vi "MicroscopeControl.vi"(0 "Microscope in":refnum<class "Microscope.lvclass">) -> (4 "Microscope Out":refnum<class "Microscope.lvclass">)   [LabVIEW 2012]
uses:
  classes/Microscope.lvclass
  typedefs/ImageEvent.ctl
  typedefs/MicroscopeEvent.ctl
  variables/GlobalUI.vi
  classes/MCCPMT.lvclass
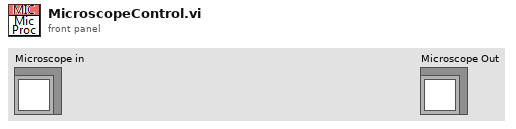
[diagram p1: front panel]
types:
  T1 = typedef "ImageEvent.ctl" = enum16{"i.Wait", "i.Acquire", "i.InitImageData", "i.ReinitImageData", "i.ReinitImageParams", "i.PreAcquire", "i.PostAcquire", "i.ClearData"}
  T2 = typedef "MicroscopeEvent.ctl" = enum16{"M.Wait", "M.RunRotation", "M.Flush", "M.Init", "M.InitStage", "M.InitImageData", "M.ReinitImageData", "M.ReinitImageParams", "M.GetSetParams", "M.InitFastHardware", "M.Pre-Acquire", "M.Acquire", "M.PostAcquire", "M.StopAcquire", "M.SetAcqStatusTrue", "M.SetAcqStatusFalse", "M.ClearImageData", "M.MoveStageDiscrete", "M.MoveStageToTarget1", "M.MoveStageToTarget2", "M.MoveStageToTarget3", "M.OpenShutters", "M.CloseShutters", "M.StartAcquireSequence", "M.ChangeParameters", "M.OpenStokes", "M.OpenPump", "M.RunSW"}
  T3 = typedef "HWsettings.ctl" = cluster{"Galvo Channels":tag, "Detector Channels":tag, "Galvo Trigger":tag, "Shutter Lines":tag[], "Max Acquisition Rate":dbl, "Recommended Acquisition Rate":dbl, "Galvo Write Rate":dbl, "Max Timebase Frequency (Hz)":dbl, "MCC Shutter Lines":refnum<k21>[], "Detector Task":refnum<k21>, "Shutter Tasks":refnum<k21>[], "Galvo Task":refnum<k21>, "Digital Image Multiplier":dbl[]}
  T4 = typedef "Scan Parameters.ctl" = cluster{"x pixels":i32, "x voltage min":dbl, "x voltage max":dbl, "y voltage min":dbl, "y voltage max":dbl, "fill frac":dbl, "Zoom":dbl, "BiDi":bool, "scan rate (ms/line)":dbl}
  T5 = typedef "Stage Parameters.ctl" = cluster{"Scan Mode":T6, "Start position mm":dbl, "End position mm":dbl, "Velocity um/sec (continuous)":dbl, "Step size microns (discrete)":dbl, "Frames to grab (grab)":i32}
  T6 = typedef "ScanMode.ctl" = enum16{"None", "Continuous", "Point Scan (CH3 cursor)", "Point Scan Move (CH3 cursor)", "Grab", "Grab Move Stage", "Grab Move Z-stage", "Cont. Move Z-stage", "Spec Move Stage", "Spec Move Cont", "Surf Calib"}
  T7 = typedef "SyncAlgo.ctl" = cluster{"Pixels/sec":dbl, "Pixel Dwell Time (us)":dbl, "Fill Factor":dbl, "Flyback Pixels":dbl, "Lines/sec":dbl, "Galvo Write rate":dbl, "Galvo Timebase divisor":i32, "total pixels per line":dbl, "Samples to Average":dbl, "Trash Samples":dbl, "Actual samples to Read per Line":dbl, "Detector Read rate":dbl, "Detector Timebase divisor":i32}
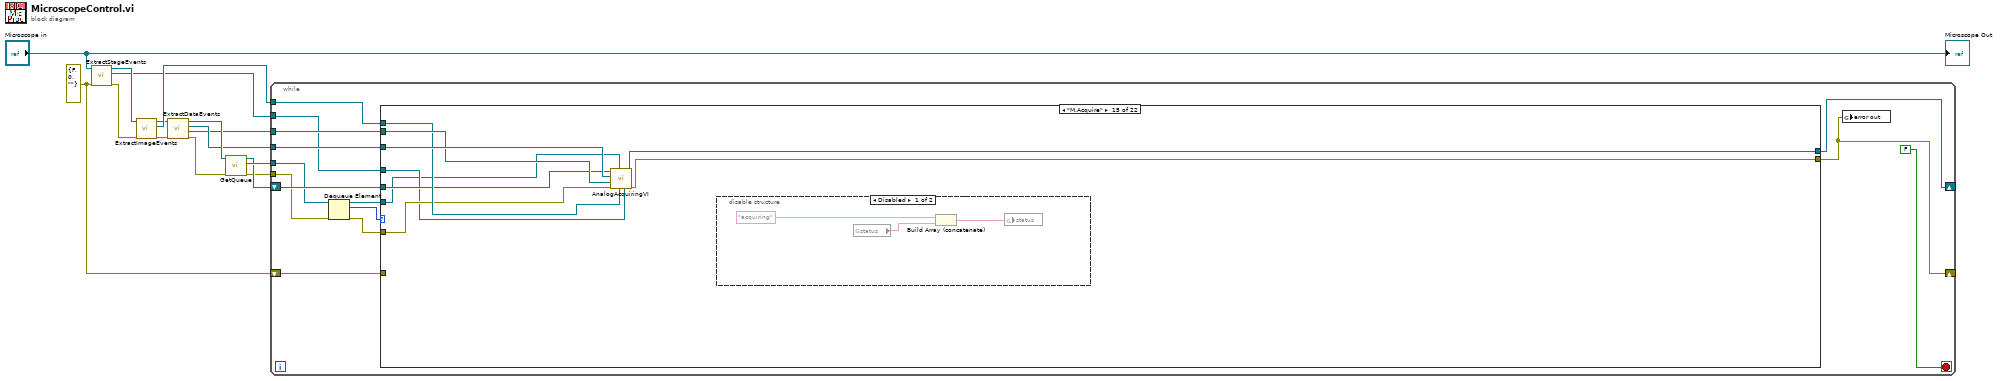
[diagram p0: block diagram]
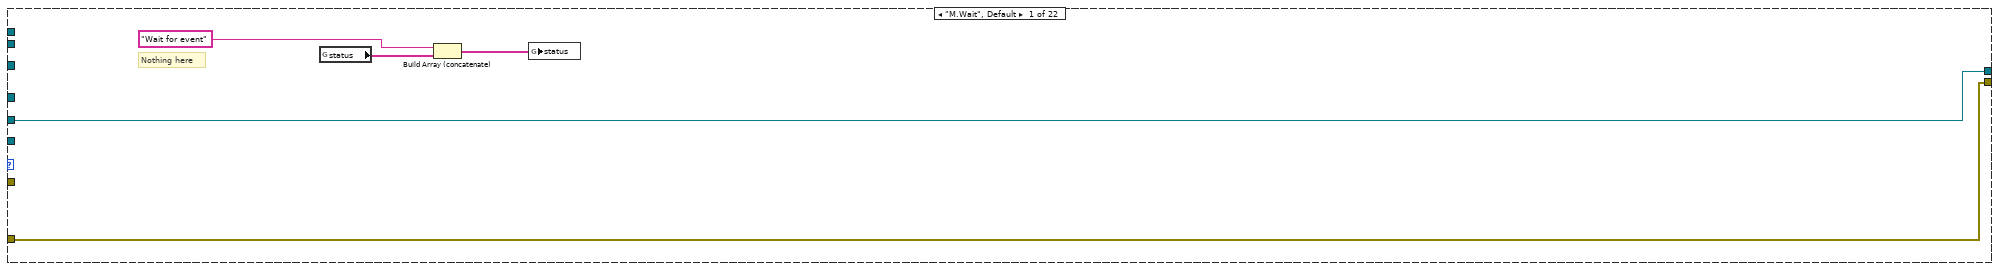
[diagram p2: hidden frame]
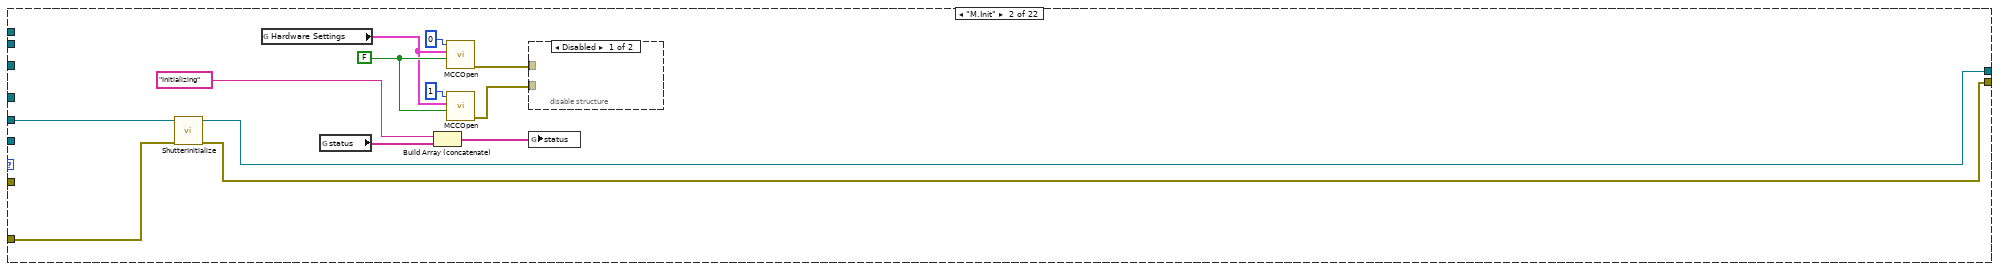
[diagram p3: hidden frame]
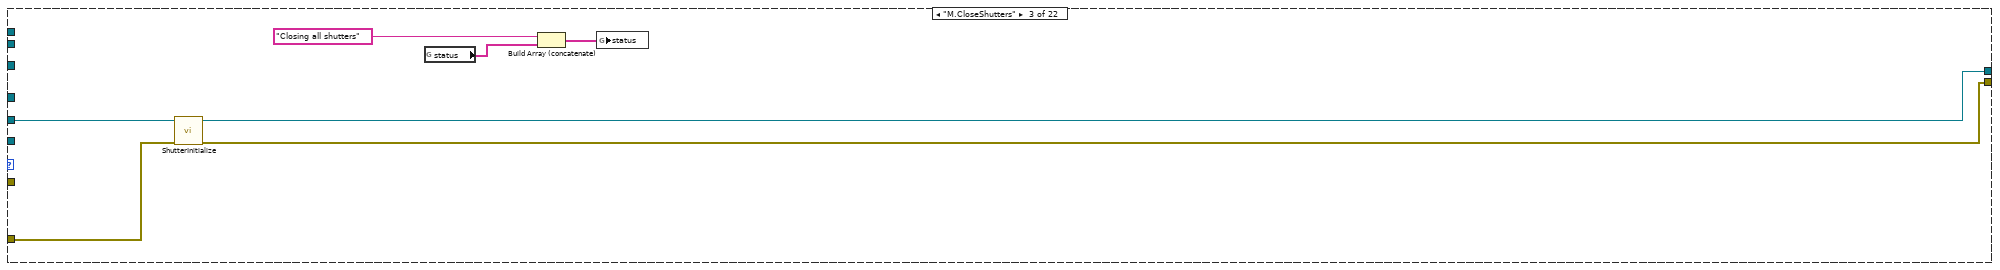
[diagram p5: hidden frame]
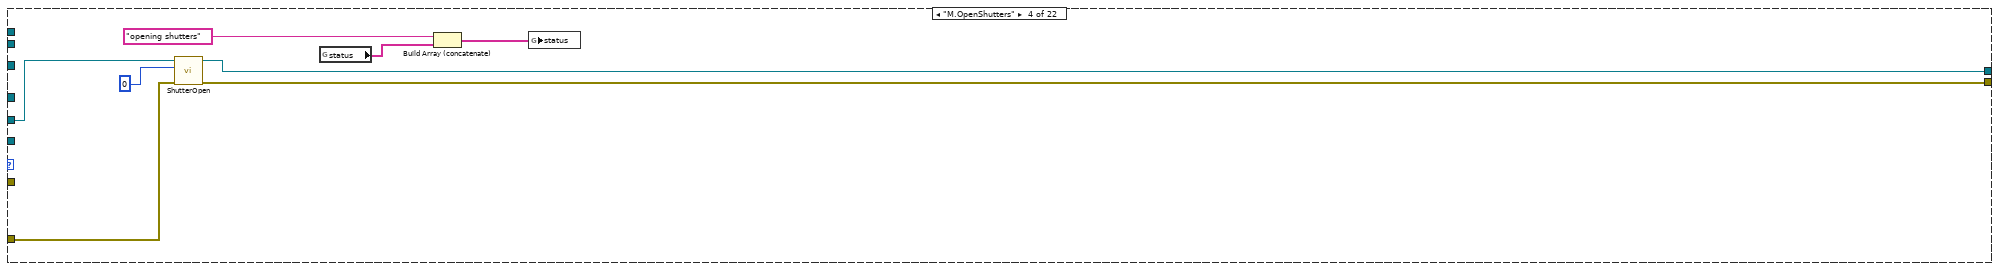
[diagram p6: hidden frame]
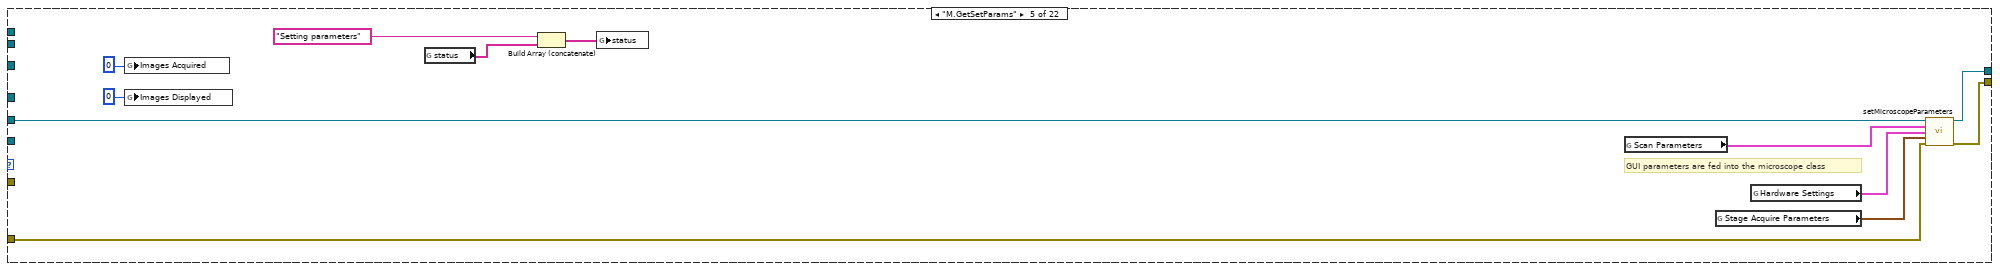
[diagram p7: hidden frame]
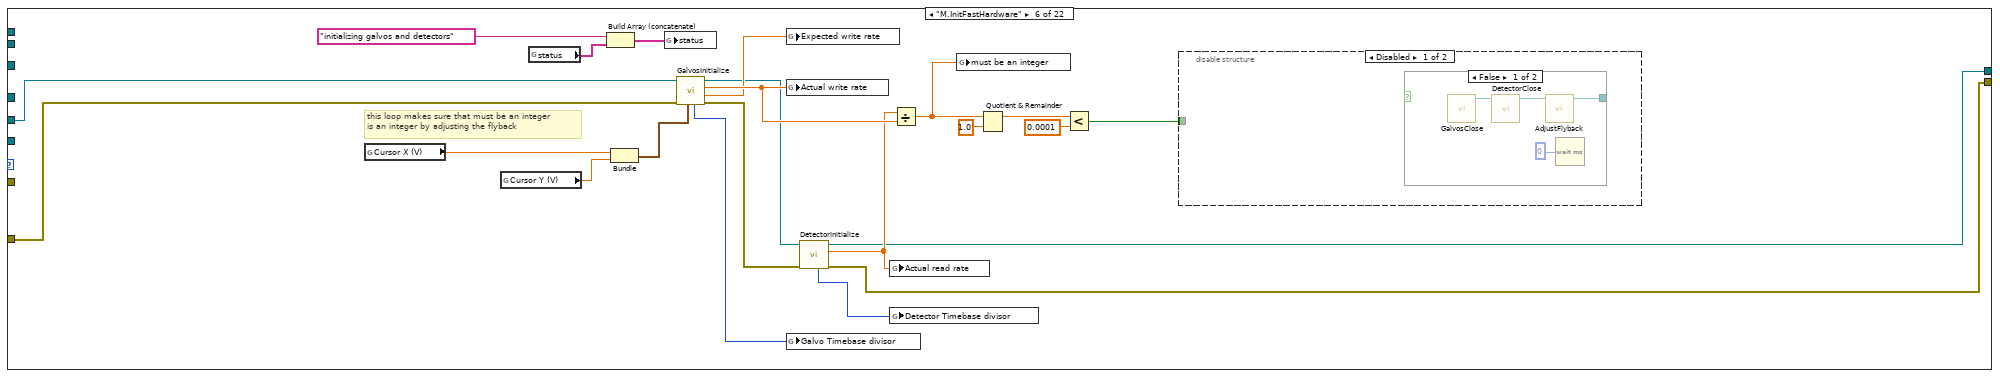
[diagram p8: hidden frame]
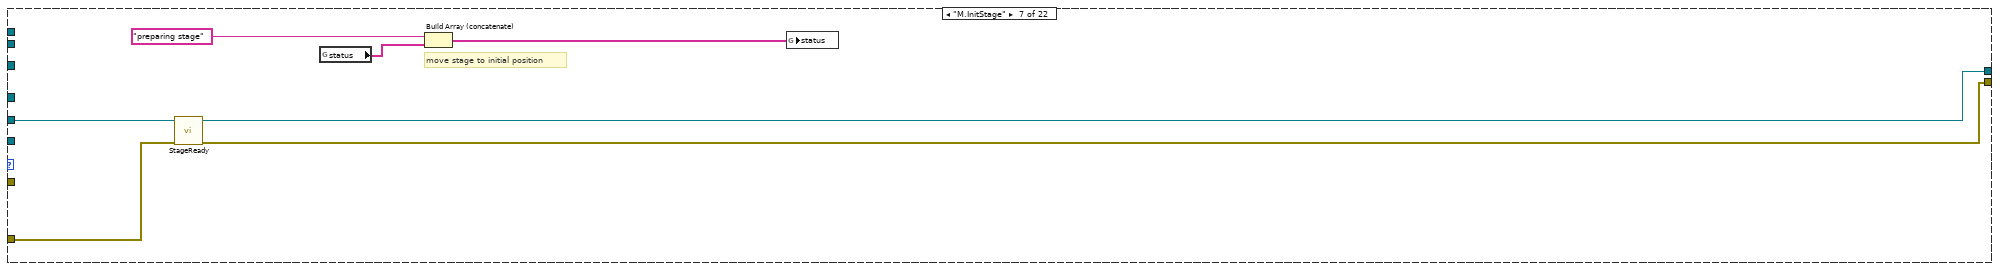
[diagram p11: hidden frame]
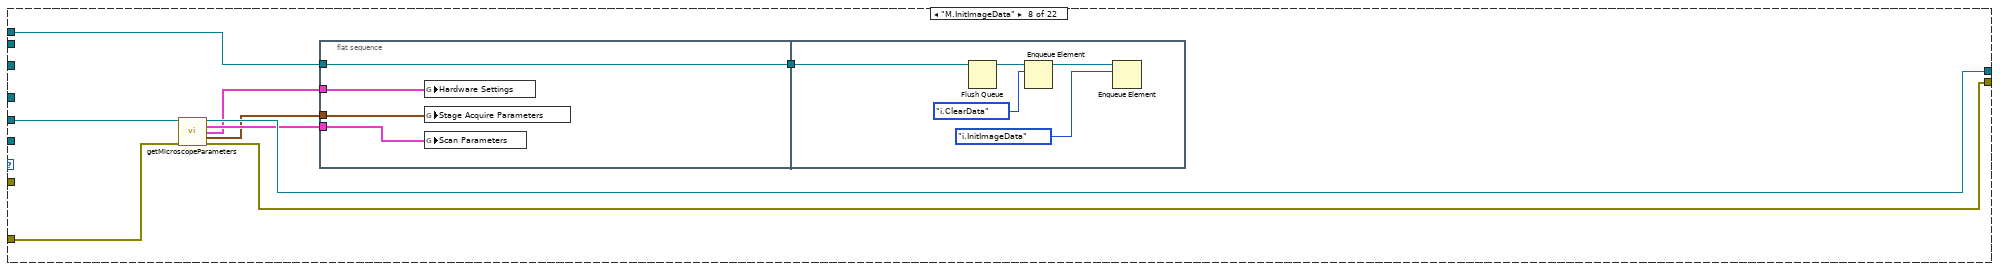
[diagram p12: hidden frame]
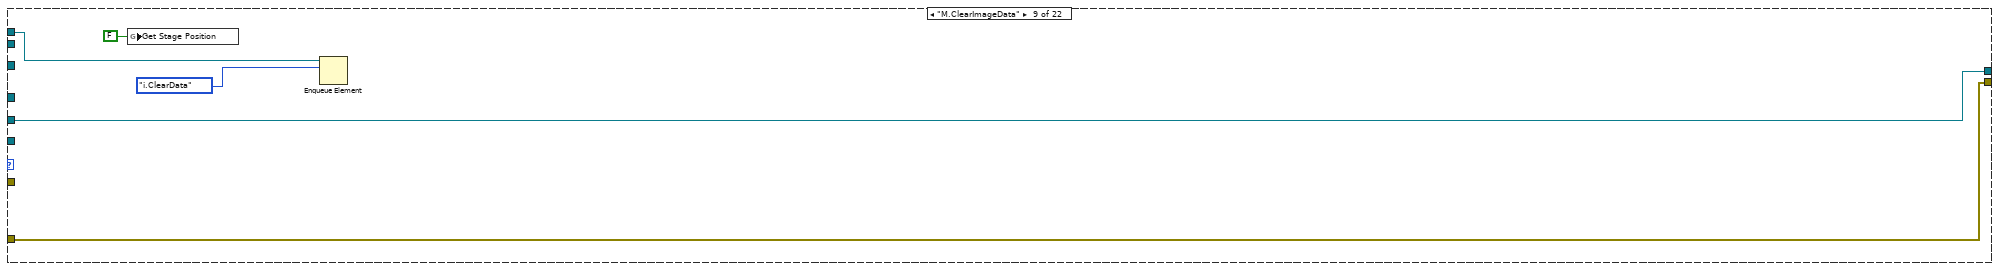
[diagram p13: hidden frame]
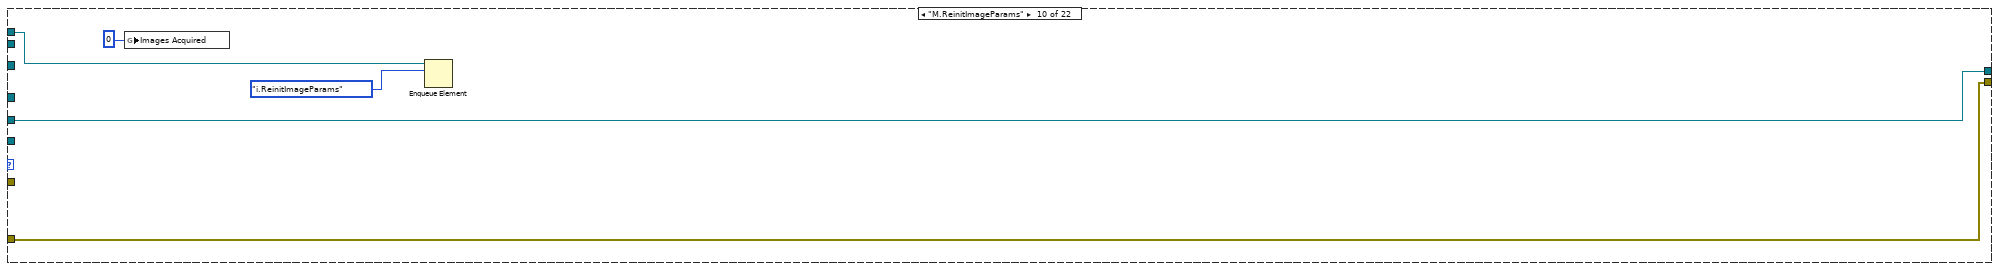
[diagram p14: hidden frame]
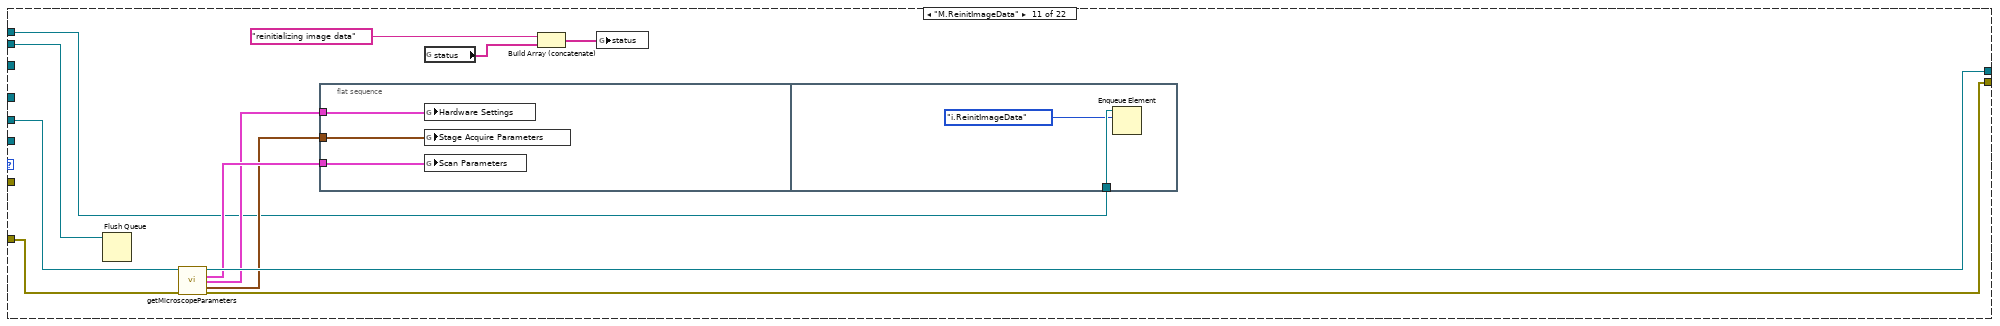
[diagram p15: hidden frame]
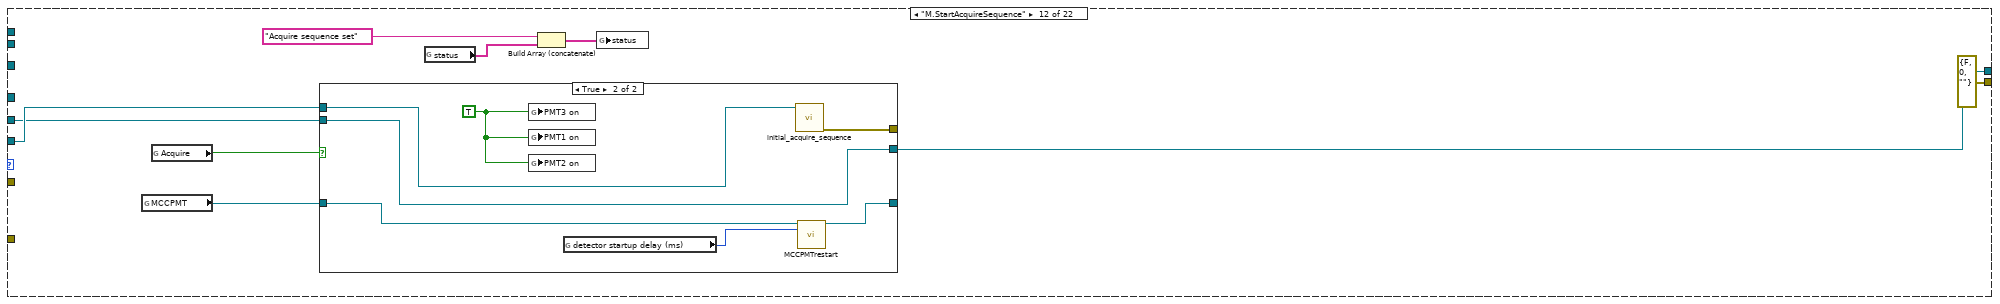
[diagram p16: hidden frame]
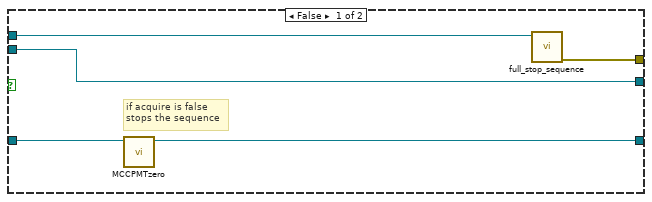
[diagram p17: hidden frame]
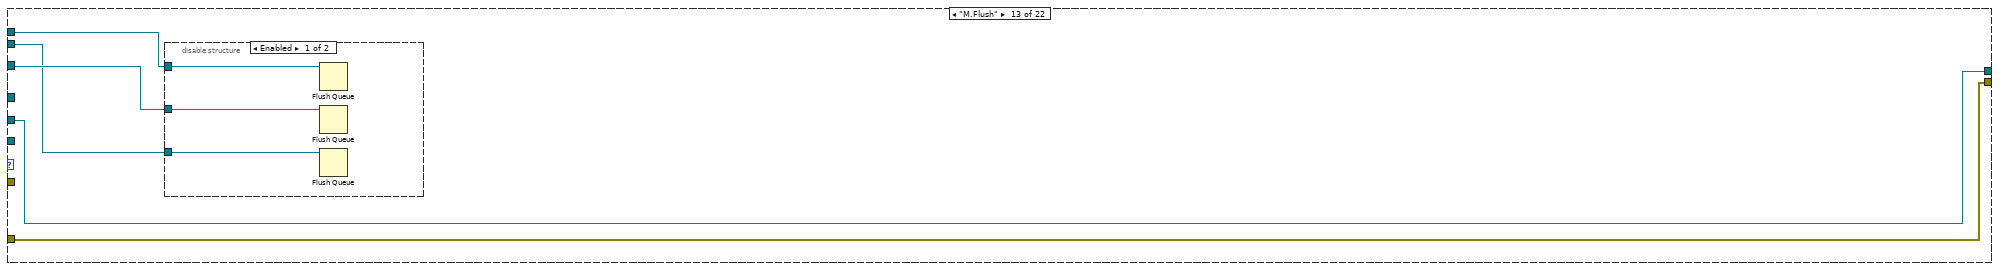
[diagram p18: hidden frame]
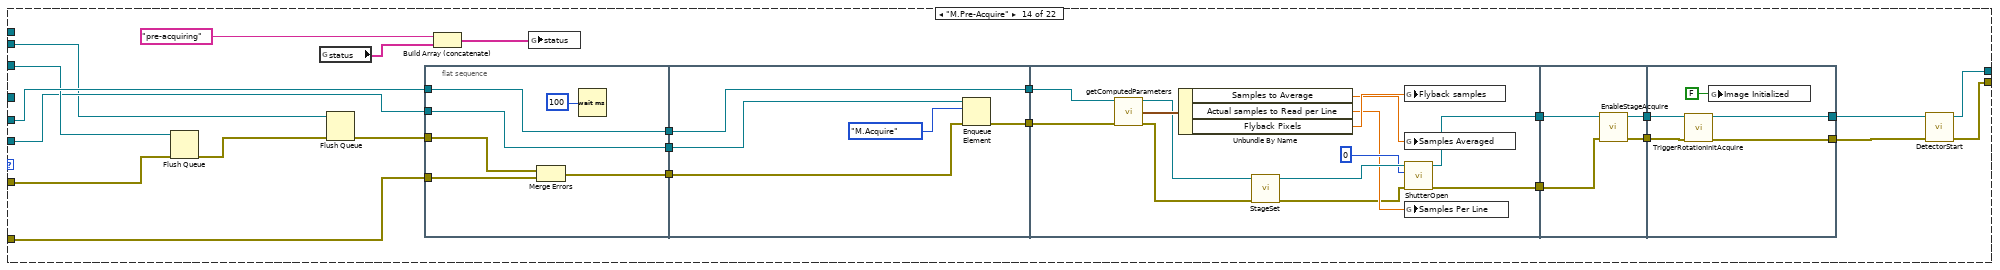
[diagram p20: hidden frame]
diagram:
  w2 = errorcluster {"status"=FALSE, "code"=0, "source"=""} ("error out")
  n1 = call "ExtractStageEvents.vi"("error in (no error)"=w2, "Microscope in"="Microscope in") -> ("error out"=w4:errorcluster, "Stage events"=w1:refnum<queue>, "Microscope out"=w5:refnum<class "Microscope.lvclass">)  [unwired: 6 in, 1 out]
  n2 = call "ExtractImageEvents.vi"("error in (no error)"=w4, "Microscope in"=w5) -> ("error out"=w6:errorcluster, "Image events"=w13:refnum<queue>, "Microscope out"=w12:refnum<class "Microscope.lvclass">)  [unwired: 7 in]
  n3 = call "ExtractDataEvents.vi"("error in (no error)"=w6, "Microscope in"=w12) -> ("error out"=w7:errorcluster, "Raw Data"=w9:refnum<queue>, "X Data"=w10:refnum<queue>, "Microscope out"=w11:refnum<class "Microscope.lvclass">)  [unwired: 6 in]
  n4 = call "GetQueue.vi"("error in (no error)"=w7, "Microscope in"=w11) -> ("error out"=w8:errorcluster, "Microscope events"=w15:refnum<queue>, "Microscope out"=w14:refnum<class "Microscope.lvclass">)  [unwired: 7 in]
  n5 = while {
    shift-right: [w28] -> _
    shift-left: w14 -> [w29]
    shift-right: [w19] -> _
    shift-left: w2 -> [w21]
    tunnel: w15 -> [w20]
    tunnel: w9 -> [w24]
    tunnel: w13 -> [w23]
    tunnel: w10 -> [w22]
    tunnel: w8 -> [w17]
    tunnel: w1 -> [w16]
    stop <- FALSE stop-if-true
    n6 = Dequeue Element(queue=w20, error in (no error)=w17) -> (queue out=w27:refnum<queue>, element=w26:T2, error out=w18:errorcluster)  [unwired: 1 in, 1 out]
    n7 = case shown="\"M.Acquire\"" w26 {
      tunnel: w29 -> [w34 w45 w52 w61 w74 w88 w103 w117 w130 w136 w148 w156 w179 w206 w245 w267 w282 w291 w299 w306 w313 w321]
      tunnel: [w34 w47 w54 w60 w64 w75 w105 w116 w130 w136 w147 w155 w179 w204 w240 w258 w269 w290 w299 w306 w309 w314] -> w28
      tunnel: [w33 w46 w53 w59 w63 w95 w104 w115 w129 w135 w145 errorcluster {"status"=FALSE, "code"=0, "source"=""} ("error out") w178 w205 w241 w257 w271 w288 w300 w307 w308 w315] -> w19
      tunnel: w21 -> [w33 w44 w51 w58 w65 w96 w102 w114 w129 w135 w146 _ w178 w203 _ w268 w280 w289 w300 w307 w312 w320]
      tunnel: w27 -> [_ _ _ _ _ _ _ _ _ _ _ w162 _ w201 w242 w264 _ _ _ _ _ _]
      tunnel: w24 -> [_ _ _ _ _ _ _ _ _ _ w140 _ w176 w200 w247 _ _ _ _ _ _ _]
      tunnel: w23 -> [_ _ _ _ _ _ _ w110 w131 w134 w141 _ w175 _ w246 w263 _ _ _ _ _ _]
      tunnel: w22 -> [_ _ _ _ _ _ _ _ _ _ _ _ w177 w202 w248 _ _ _ _ _ _ _]
      tunnel: w18 -> [_ _ _ _ _ _ _ _ _ _ _ _ _ w192 w244 _ _ _ _ _ _ _]
      tunnel: w16 -> [_ _ _ _ _ _ _ _ _ _ _ _ _ _ w243 _ w270 _ _ _ _ _]
      frame "M.Wait", Default {
        # "Nothing here"
        n8 = global read "GlobalUI.vi" "status"() -> (w32:string[])
        n9 = Build Array (concatenate)("Wait for event" ("status"), w32) -> (w31:string[])
        n10 = global write "GlobalUI.vi" "status"(w31) -> ()
      }
      frame "M.Init" {
        w41 = FALSE ("Open")
        n11 = call "ShutterInitialize.vi"("error in (no error)"=w44, "Microscope in"=w45) -> ("error out"=w46:errorcluster, "Microscope out"=w47:refnum<class "Microscope.lvclass">)  [unwired: 8 in]
        n12 = global read "GlobalUI.vi" "Hardware Settings"() -> (w37:T3)
        n13 = global read "GlobalUI.vi" "status"() -> (w40:string[])
        n14 = Build Array (concatenate)("Initializing" ("status"), w40) -> (w39:string[])
        n15 = call "MCCOpen.vi"("Open"=w41, "Hardware Settings"=w37, "index"=0) -> ("error out"=w36:errorcluster)  [unwired: 8 in]
        n16 = call "MCCOpen.vi"("Open"=w41, "Hardware Settings"=w37, "index"=1) -> ("error out"=w35:errorcluster)  [unwired: 8 in]
        n17 = disable-structure shown="Disabled" {
          disable-tunnel: w36 -> [_ _]
          disable-tunnel: w35 -> [_ _]
          frame Disabled {
          }
          frame Enabled {
          }
        }
        n18 = global write "GlobalUI.vi" "status"(w39) -> ()
      }
      frame "M.CloseShutters" {
        n19 = call "ShutterInitialize.vi"("error in (no error)"=w51, "Microscope in"=w52) -> ("error out"=w53:errorcluster, "Microscope out"=w54:refnum<class "Microscope.lvclass">)  [unwired: 8 in]
        n20 = global read "GlobalUI.vi" "status"() -> (w50:string[])
        n21 = Build Array (concatenate)("Closing all shutters" ("status"), w50) -> (w48:string[])
        n22 = global write "GlobalUI.vi" "status"(w48) -> ()
      }
      frame "M.OpenShutters" {
        n23 = call "ShutterOpen.vi"("error in (no error)"=w58, "Shutter number"=0, "Microscope in"=w61) -> ("error out"=w59:errorcluster, "Microscope out"=w60:refnum<class "Microscope.lvclass">)  [unwired: 7 in]
        n24 = global read "GlobalUI.vi" "status"() -> (w57:string[])
        n25 = Build Array (concatenate)("opening shutters" ("status"), w57) -> (w56:string[])
        n26 = global write "GlobalUI.vi" "status"(w56) -> ()
      }
      frame "M.GetSetParams" {
        # "GUI parameters are fed into the microscope class"
        n27 = global write "GlobalUI.vi" "Images Acquired"(0 ("images grabbed")) -> ()
        n28 = global write "GlobalUI.vi" "Images Displayed"(0 ("Frames grabbed")) -> ()
        n29 = global read "GlobalUI.vi" "status"() -> (w69:string[])
        n30 = Build Array (concatenate)("Setting parameters" ("status"), w69) -> (w68:string[])
        n31 = global write "GlobalUI.vi" "status"(w68) -> ()
        n32 = global read "GlobalUI.vi" "Scan Parameters"() -> (w67:T4)
        n33 = global read "GlobalUI.vi" "Stage Acquire Parameters"() -> (w70:T5)
        n34 = global read "GlobalUI.vi" "Hardware Settings"() -> (w66:T3)
        n35 = call "setMicroscopeParameters.vi"("Microscope in"=w74, "Scan Parameters"=w67, "Hardware Settings"=w66, "Stage Acquire Parameters"=w70, "error in (no error)"=w65) -> ("Microscope out"=w64:refnum<class "Microscope.lvclass">, "error out"=w63:errorcluster)  [unwired: 9 in]
      }
      frame "M.InitFastHardware" {
        # "this loop makes sure that must be an integer\nis an integer by adjusting the flyback"
        n36 = global read "GlobalUI.vi" "Cursor X (V)"() -> (w91:dbl)
        n37 = global read "GlobalUI.vi" "Cursor Y (V)"() -> (w90:dbl)
        n38 = global read "GlobalUI.vi" "status"() -> (w94:string[])
        n39 = Build Array (concatenate)("initializing galvos and detectors" ("status"), w94) -> (w93:string[])
        n40 = Bundle("Cursor X (V)"=w91, "Cursor Y (V)"=w90) -> (w89:cluster{"Cursor X (V)":dbl, "Cursor Y (V)":dbl})  [unwired: 1 in]
        n41 = global write "GlobalUI.vi" "status"(w93) -> ()
        n42 = call "GalvosInitialize.vi"("Cursor Position (V)"=w89, "error in (no error)"=w96, "Microscope in"=w88) -> ("error out"=w87:errorcluster, "Galvo Write Rate"=w85:dbl, "actual write rate"=w86:dbl, "Microscope out"=w83:refnum<class "Microscope.lvclass">, "Galvo Timebase divisor"=w84:i32)  [unwired: 4 in]
        n43 = global write "GlobalUI.vi" "Expected write rate"(w85) -> ()
        n44 = global write "GlobalUI.vi" "Actual write rate"(w86) -> ()
        n45 = global write "GlobalUI.vi" "Galvo Timebase divisor"(w84) -> ()
        n46 = call "DetectorInitialize.vi"("error in (no error)"=w87, "Microscope in"=w83) -> ("error out"=w95:errorcluster, "Actual read rate"=w82:dbl, "Microscope out"=w75:refnum<class "Microscope.lvclass">, "Detector Timebase divisor"=w81:i32)  [unwired: 6 in]
        n47 = global write "GlobalUI.vi" "Actual read rate"(w82) -> ()
        n48 = global write "GlobalUI.vi" "Detector Timebase divisor"(w81) -> ()
        n49 = Divide(x=w82, y=w86) -> (x/y=w80:dbl)
        n50 = global write "GlobalUI.vi" "must be an integer"(w80) -> ()
        n51 = Quotient & Remainder(x=w80, y=1.0) -> (x-y*floor(x/y)=w77:dbl)  [unwired: 1 out]
        n52 = Less?(x=w77, y=0.0001) -> (x < y?=w76:bool)
        n53 = disable-structure shown="Disabled" {
          disable-tunnel: w76 -> [w97 _]
          frame Disabled {
            n54 = case shown="False" {
              selector: _ -> [_ _]
              tunnel: [w98 _] -> _
              frame False {
                n55 = call "GalvosClose.vi"() -> ("Microscope out"=w99:refnum<class "Microscope.lvclass">)  [unwired: 10 in, 1 out]
                n56 = call "DetectorClose.vi"("Microscope in"=w99) -> ("Microscope out"=w101:refnum<class "Microscope.lvclass">)  [unwired: 9 in, 1 out]
                n57 = call "AdjustFlyback.vi"("Microscope in"=w101) -> ("Microscope out"=w98:refnum<class "Microscope.lvclass">)  [unwired: 9 in, 1 out]
                n58 = Wait (ms)(milliseconds to wait=u32 0) -> ()  [unwired: 1 out]
              }
              frame True {
              }
            }
          }
          frame Enabled {
          }
        }
      }
      frame "M.InitStage" {
        # "move stage to initial position"
        n59 = call "StageReady.vi"("error in (no error)"=w102, "Microscope in"=w103) -> ("error out"=w104:errorcluster, "Microscope out"=w105:refnum<class "Microscope.lvclass">)  [unwired: 8 in]
        n60 = global read "GlobalUI.vi" "status"() -> (w107:string[])
        n61 = Build Array (concatenate)("preparing stage" ("status"), w107) -> (w108:string[])
        n62 = global write "GlobalUI.vi" "status"(w108) -> ()
      }
      frame "M.InitImageData" {
        n63 = call "getMicroscopeParameters.vi"("Microscope in"=w117, "error in (no error)"=w114) -> ("Microscope out"=w116:refnum<class "Microscope.lvclass">, "Scan Parameters"=w113:T4, "Hardware Settings"=w112:T3, "Stage Acquire Parameters"=w111:T5, "error out"=w115:errorcluster)  [unwired: 9 in]
        n64 = flat-sequence {
          tunnel: w113 -> [w119]
          tunnel: w112 -> [w120]
          tunnel: w111 -> [w118]
          tunnel: w110 -> [w121]
          tunnel: [w121] -> w109
          tunnel: w109 -> [w125]
          frame #0 {
            n65 = global write "GlobalUI.vi" "Hardware Settings"(w120) -> ()
            n66 = global write "GlobalUI.vi" "Stage Acquire Parameters"(w118) -> ()
            n67 = global write "GlobalUI.vi" "Scan Parameters"(w119) -> ()
          }
          frame #1 {
            n68 = Flush Queue(queue=w125) -> (queue out=w124:refnum<queue>)  [unwired: 1 in, 2 out]
            n69 = Enqueue Element(queue=w124, element=ImageEvent."i.ClearData") -> (queue out=w123:refnum<queue>)  [unwired: 2 in, 2 out]
            n70 = Enqueue Element(queue=w123, element=ImageEvent."i.InitImageData") -> ()  [unwired: 2 in, 3 out]
          }
        }
      }
      frame "M.ClearImageData" {
        n71 = global write "GlobalUI.vi" "Get Stage Position"(FALSE ("Get Stage Position")) -> ()
        n72 = Enqueue Element(queue=w131, element=ImageEvent."i.ClearData") -> ()  [unwired: 2 in, 3 out]
      }
      frame "M.ReinitImageParams" {
        n73 = global write "GlobalUI.vi" "Images Acquired"(0 ("Dgrabbed")) -> ()
        n74 = Enqueue Element(queue=w134, element=ImageEvent."i.ReinitImageParams") -> ()  [unwired: 2 in, 3 out]
      }
      frame "M.ReinitImageData" {
        n75 = Flush Queue(queue=w140) -> ()  [unwired: 1 in, 3 out]
        n76 = call "getMicroscopeParameters.vi"("Microscope in"=w148, "error in (no error)"=w146) -> ("Microscope out"=w147:refnum<class "Microscope.lvclass">, "Scan Parameters"=w144:T4, "Hardware Settings"=w143:T3, "Stage Acquire Parameters"=w142:T5, "error out"=w145:errorcluster)  [unwired: 9 in]
        n77 = flat-sequence {
          tunnel: w144 -> [w150]
          tunnel: w143 -> [w151]
          tunnel: w142 -> [w149]
          tunnel: w141 -> [w153]
          frame #0 {
            n78 = global write "GlobalUI.vi" "Hardware Settings"(w151) -> ()
            n79 = global write "GlobalUI.vi" "Stage Acquire Parameters"(w149) -> ()
            n80 = global write "GlobalUI.vi" "Scan Parameters"(w150) -> ()
          }
          frame #1 {
            n81 = Enqueue Element(queue=w153, element=ImageEvent."i.ReinitImageData") -> ()  [unwired: 2 in, 3 out]
          }
        }
        n82 = global read "GlobalUI.vi" "status"() -> (w139:string[])
        n83 = Build Array (concatenate)("reinitializing image data" ("status"), w139) -> (w138:string[])
        n84 = global write "GlobalUI.vi" "status"(w138) -> ()
      }
      frame "M.StartAcquireSequence" {
        n85 = global read "GlobalUI.vi" "MCCPMT"() -> (w157:refnum<class "MCCPMT.lvclass">)
        n86 = global read "GlobalUI.vi" "Acquire"() -> (w158:bool)
        n87 = case shown="True" w158 {
          tunnel: [w167 w174] -> _
          tunnel: [w166 w173] -> _
          tunnel: w157 -> [w165 w172]
          tunnel: w162 -> [w164 w168]
          tunnel: w156 -> [w163 w169]
          tunnel: [w163 w169] -> w155
          frame False {
            # "if acquire is false\nstops the sequence"
            n88 = call "MCCPMTzero.vi"("MCCPMT in"=w165) -> ("MCCPMT out"=w166:refnum<class "MCCPMT.lvclass">)  [unwired: 9 in, 1 out]
            n89 = call "full_stop_sequence.vi"("Queue in"=w164) -> ("error out"=w167:errorcluster)  [unwired: 9 in, 1 out]
          }
          frame True {
            w171 = TRUE ("PMT2 on")
            n90 = global write "GlobalUI.vi" "PMT3 on"(w171) -> ()
            n91 = global write "GlobalUI.vi" "PMT1 on"(w171) -> ()
            n92 = global write "GlobalUI.vi" "PMT2 on"(w171) -> ()
            n93 = global read "GlobalUI.vi" "detector startup delay (ms)"() -> (w170:u32)
            n94 = call "initial_acquire_sequence.vi"("Queue in"=w168) -> ("error out"=w174:errorcluster)  [unwired: 9 in, 1 out]
            n95 = call "MCCPMTrestart.vi"("MCCPMT in"=w172, "milliseconds to wait"=w170) -> ("MCCPMT out"=w173:refnum<class "MCCPMT.lvclass">)  [unwired: 9 in, 4 out]
          }
        }
        n96 = global read "GlobalUI.vi" "status"() -> (w161:string[])
        n97 = Build Array (concatenate)("Acquire sequence set" ("status"), w161) -> (w159:string[])
        n98 = global write "GlobalUI.vi" "status"(w159) -> ()
      }
      frame "M.Flush" {
        n99 = disable-structure shown="Enabled" {
          disable-tunnel: w177 -> [w182 _]
          disable-tunnel: w176 -> [w181 _]
          disable-tunnel: w175 -> [w180 _]
          frame Enabled {
            n100 = Flush Queue(queue=w180) -> ()  [unwired: 1 in, 3 out]
            n101 = Flush Queue(queue=w182) -> ()  [unwired: 1 in, 3 out]
            n102 = Flush Queue(queue=w181) -> ()  [unwired: 1 in, 3 out]
          }
          frame Disabled {
          }
        }
      }
      frame "M.Pre-Acquire" {
        n103 = Flush Queue(queue=w202, error in (no error)=w192) -> (error out=w193:errorcluster)  [unwired: 2 out]
        n104 = global read "GlobalUI.vi" "status"() -> (w199:string[])
        n105 = Flush Queue(queue=w200, error in (no error)=w193) -> (error out=w194:errorcluster)  [unwired: 2 out]
        n106 = flat-sequence {
          tunnel: w206 -> [w212]
          tunnel: [w212] -> w191
          tunnel: w203 -> [w208]
          tunnel: w201 -> [w211]
          tunnel: [w211] -> w190
          tunnel: w194 -> [w209]
          tunnel: [w207] -> w189
          tunnel: w191 -> [w214]
          tunnel: [w214] -> w188
          tunnel: [w213] -> w187
          tunnel: w190 -> [w217]
          tunnel: w189 -> [w215]
          tunnel: w188 -> [w222]
          tunnel: [w227] -> w186
          tunnel: w187 -> [w221]
          tunnel: [w226] -> w185
          tunnel: w186 -> [w232]
          tunnel: w185 -> [w234]
          tunnel: [w233] -> w184
          tunnel: [w231] -> w183
          tunnel: [w237] -> w196
          tunnel: [w235] -> w195
          tunnel: w184 -> [w238]
          tunnel: w183 -> [w236]
          frame #0 {
            n107 = Merge Errors(w209, w208) -> (w207:errorcluster)
            n108 = Wait (ms)(milliseconds to wait=u32 100) -> ()  [unwired: 1 out]
          }
          frame #1 {
            n109 = Enqueue Element(queue=w217, element=MicroscopeEvent."M.Acquire", error in (no error)=w215) -> (error out=w213:errorcluster)  [unwired: 1 in, 2 out]
          }
          frame #2 {
            n110 = call "getComputedParameters.vi"("Microscope in"=w222, "error in (no error)"=w221) -> ("Microscope out"=w220:refnum<class "Microscope.lvclass">, "Computed Parameters"=w228:T7, "error out"=w219:errorcluster)  [unwired: 10 in, 1 out]
            n111 = Unbundle By Name(w228) -> ("Samples to Average"=w223:dbl, "Actual samples to Read per Line"=w224:dbl, "Flyback Pixels"=w225:dbl)
            n112 = call "StageSet.vi"("error in (no error)"=w219, "Microscope in"=w220) -> ("error out"=w218:errorcluster, "Microscope out"=w230:refnum<class "Microscope.lvclass">)  [unwired: 8 in]
            n113 = global write "GlobalUI.vi" "Flyback samples"(w225) -> ()
            n114 = global write "GlobalUI.vi" "Samples Averaged"(w223) -> ()
            n115 = call "ShutterOpen.vi"("error in (no error)"=w218, "Shutter number"=0, "Microscope in"=w230) -> ("error out"=w227:errorcluster, "Microscope out"=w226:refnum<class "Microscope.lvclass">)  [unwired: 7 in]
            n116 = global write "GlobalUI.vi" "Samples Per Line"(w224) -> ()
          }
          frame #3 {
            n117 = call "EnableStageAcquire.vi"("error in (no error)"=w232, "Microscope in"=w234) -> ("error out"=w231:errorcluster, "Microscope out"=w233:refnum<class "Microscope.lvclass">)  [unwired: 8 in]
          }
          frame #4 {
            n118 = call "TriggerRotationInitAcquire.vi"("Microscope in"=w238, "error in (no error)"=w236) -> ("Microscope out"=w237:refnum<class "Microscope.lvclass">, "error out"=w235:errorcluster)  [unwired: 12 in]
            n119 = global write "GlobalUI.vi" "Image Initialized"(FALSE ("Image Initialized")) -> ()
          }
        }
        n120 = Build Array (concatenate)("pre-acquiring" ("status"), w199) -> (w197:string[])
        n121 = global write "GlobalUI.vi" "status"(w197) -> ()
        n122 = call "DetectorStart.vi"("error in (no error)"=w195, "Microscope in"=w196) -> ("error out"=w205:errorcluster, "Microscope out"=w204:refnum<class "Microscope.lvclass">)  [unwired: 8 in]
      }
      frame "M.Acquire" {
        n123 = call "AnalogAcquiringVI.vi"("Stage events"=w243, "Image events"=w246, "Microscope events"=w242, "error in (no error)"=w244, "raw data"=w247, "X Data"=w248, "Microscope in"=w245) -> ("error out"=w241:errorcluster, "Microscope out"=w240:refnum<class "Microscope.lvclass">)  [unwired: 3 in]
        n124 = disable-structure shown="Disabled" {
          frame Disabled {
            n125 = global read "GlobalUI.vi" "status"() -> (w251:string[])
            n126 = Build Array (concatenate)("acquiring" ("status"), w251) -> (w250:string[])
            n127 = global write "GlobalUI.vi" "status"(w250) -> ()
          }
          frame Enabled {
          }
        }
      }
      frame "M.PostAcquire" {
        n128 = global read "GlobalUI.vi" "status"() -> (w262:string[])
        n129 = Build Array (concatenate)("post acquire" ("status"), w262) -> (w261:string[])
        n130 = global write "GlobalUI.vi" "status"(w261) -> ()
        n131 = global read "GlobalUI.vi" "Acquire"() -> (w259:bool)
        n132 = call "setreinitMicroscope.vi"("Microscope in"=w267, "microscope event queue"=w264, "image event queue"=w263, "error in (no error)"=w268, "acquire?"=w259) -> ("Microscope out"=w266:refnum<class "Microscope.lvclass">, "error out"=w265:errorcluster)  [unwired: 1 in]
        n133 = call "DetectorClose.vi"("error in (no error)"=w265, "Microscope in"=w266) -> ("error out"=w254:errorcluster, "Microscope out"=w255:refnum<class "Microscope.lvclass">)  [unwired: 8 in]
        n134 = call "Command.vi"("error in (no error)"=w254, "Microscope events"=MicroscopeEvent."M.ClearImageData", "Microscope in"=w255) -> ("error out"=w252:errorcluster, "Microscope out"=w256:refnum<class "Microscope.lvclass">)  [unwired: 7 in]
        n135 = call "GalvosClose.vi"("error in (no error)"=w252, "Microscope in"=w256) -> ("error out"=w257:errorcluster, "Microscope out"=w258:refnum<class "Microscope.lvclass">)  [unwired: 8 in]
      }
      frame "M.StopAcquire" {
        w273 = FALSE ("get position?")
        w274 = FALSE ("PMT2 on")
        n136 = global read "GlobalUI.vi" "MCCPMT"() -> (w276:refnum<class "MCCPMT.lvclass">)
        n137 = global write "GlobalUI.vi" "PMT3 on"(w274) -> ()
        n138 = global write "GlobalUI.vi" "PMT1 on"(w274) -> ()
        n139 = global write "GlobalUI.vi" "PMT2 on"(w274) -> ()
        n140 = global write "GlobalUI.vi" "Get Stage Position"(w273) -> ()
        n141 = global write "GlobalUI.vi" "Autosave"(w273) -> ()
        n142 = call "ShutterInitialize.vi"("error in (no error)"=w280, "Microscope in"=w282) -> ("error out"=w272:errorcluster, "Microscope out"=w281:refnum<class "Microscope.lvclass">)  [unwired: 8 in]
        n143 = call "MCCPMTzero.vi"("MCCPMT in"=w276) -> ("MCCPMT out"=w275:refnum<class "MCCPMT.lvclass">)  [unwired: 9 in, 1 out]
        n144 = call "StageStopMove.vi"("error in (no error)"=w272, "Stage events"=w270, "Microscope in"=w281) -> ("error out"=w271:errorcluster, "Microscope out"=w269:refnum<class "Microscope.lvclass">)  [unwired: 7 in]
        n145 = global write "GlobalUI.vi" "MCCPMT"(w275) -> ()
        n146 = global read "GlobalUI.vi" "status"() -> (w279:string[])
        n147 = Build Array (concatenate)("stopping acquisition" ("status"), w279) -> (w277:string[])
        n148 = call "DetectorClose.vi"("Microscope in"=w269) -> ()  [unwired: 9 in, 2 out]
        n149 = call "GalvosClose.vi"("Microscope in"=w269) -> ()  [unwired: 9 in, 2 out]
        n150 = global write "GlobalUI.vi" "status"(w277) -> ()
      }
      frame "M.MoveStageDiscrete" {
        n151 = global read "GlobalUI.vi" "status"() -> (w287:string[])
        n152 = Build Array (concatenate)("moving stage (discrete)" ("status"), w287) -> (w286:string[])
        n153 = global write "GlobalUI.vi" "status"(w286) -> ()
        n154 = global read "GlobalUI.vi" "Acquire"() -> (w284:bool)
        n155 = call "StageMoveDiscrete.vi"("time delay before acquisition (ms)"=u32 2000, "error in (no error)"=w289, "acquire?"=w284, "Microscope in"=w291) -> ("error out"=w288:errorcluster, "Microscope out"=w290:refnum<class "Microscope.lvclass">)  [unwired: 6 in]
      }
      frame "M.SetAcqStatusTrue" {
        n156 = global write "GlobalUI.vi" "Acquire"(TRUE ("Stage Acquire")) -> ()
        n157 = global read "GlobalUI.vi" "Scan Parameters"() -> (w295:T4)
        n158 = global read "GlobalUI.vi" "Zoom"() -> (w293:dbl)
        n159 = global read "GlobalUI.vi" "status"() -> (w298:string[])
        n160 = Bundle By Name(cluster=w295, "Zoom"=w293) -> (w294:T4)
        n161 = Build Array (concatenate)("enabling acquire buttons" ("status"), w298) -> (w297:string[])
        n162 = global write "GlobalUI.vi" "Scan Parameters"(w294) -> ()
        n163 = global write "GlobalUI.vi" "status"(w297) -> ()
      }
      frame "M.SetAcqStatusFalse" {
        n164 = global write "GlobalUI.vi" "MakeAcquireButtonFalse"(TRUE ("Stage Acquire")) -> ()
        n165 = global write "GlobalUI.vi" "Acquire"(FALSE ("Stage Acquire")) -> ()
        n166 = global read "GlobalUI.vi" "status"() -> (w305:string[])
        n167 = Build Array (concatenate)("Setting acquire button to false" ("status"), w305) -> (w304:string[])
        n168 = global write "GlobalUI.vi" "status"(w304) -> ()
      }
      frame "M.RunSW" {
        n169 = call "CallerRunSpectraWiz.vi"("error in (no error)"=w312, "Microscope in"=w313) -> ("error out"=w310:errorcluster, "Microscope out"=w311:refnum<class "Microscope.lvclass">)  [unwired: 8 in]
        n170 = call "TriggerSpectraWizInit.vi"("error in (no error)"=w310, "Microscope in"=w311) -> ("error out"=w308:errorcluster, "Microscope out"=w309:refnum<class "Microscope.lvclass">)  [unwired: 8 in]
      }
      frame "M.RunRotation" {
        n171 = call "CallerRunRotation.vi"("error in (no error)"=w320, "Microscope in"=w321) -> ("error out"=w318:errorcluster, "Microscope out"=w319:refnum<class "Microscope.lvclass">)  [unwired: 8 in]
        n172 = call "TriggerRotationInit.vi"("Microscope in"=w319, "error in (no error)"=w318) -> ("Microscope out"=w317:refnum<class "Microscope.lvclass">, "error out"=w316:errorcluster)  [unwired: 12 in]
        n173 = flat-sequence {
          tunnel: w317 -> [w325]
          tunnel: w316 -> [w324]
          tunnel: [w325] -> w314
          tunnel: [w324] -> w315
          frame #0 {
            n174 = global write "GlobalUI.vi" "Rotation Acquire Ready?"(TRUE ("Rotation Acquire Ready?")) -> ()
            n175 = Wait (ms)(milliseconds to wait=u32 100) -> ()  [unwired: 1 out]
          }
        }
      }
    }
    n176 = global write "GlobalUI.vi" "error out"(w19) -> ()
  }
  "Microscope Out" <- "Microscope in"
